vi "water_level_UI.vi"() -> ()   [LabVIEW 2020]
panel:
  out "Water level status":dbl(slide) scale=0.0..100.0
  in  "VISA resource name":refnum<visa-resource-name>
  in  "Table Control":string[][](table)
  out "Water level status":dbl(graph)
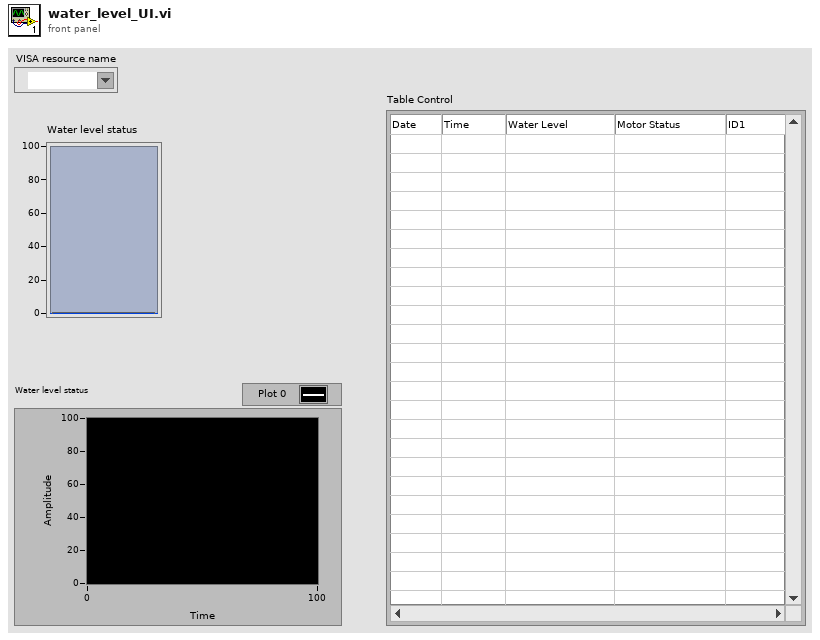
[diagram p1: front panel]
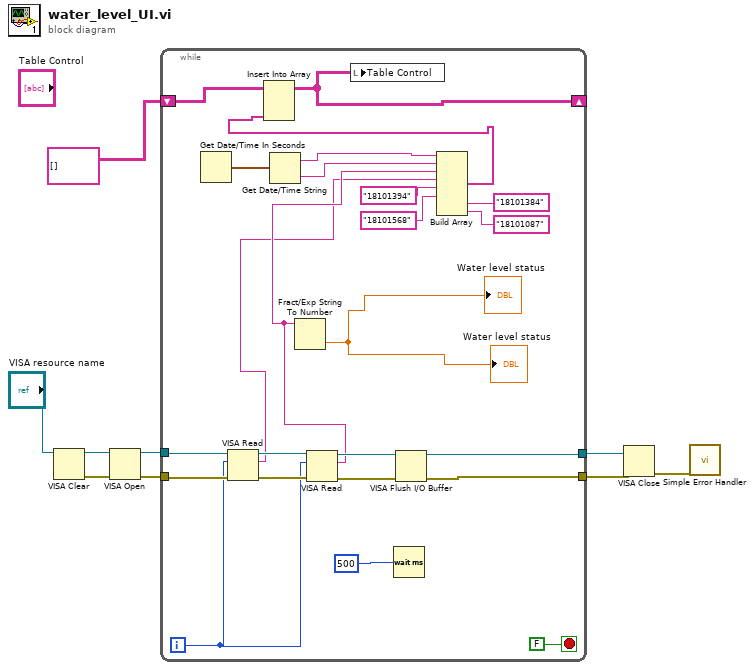
[diagram p0: block diagram]
diagram:
  n1 = VISA Clear(VISA resource name="VISA resource name") -> (VISA resource name out=w9:refnum<visa-resource-name>, error out=w8:errorcluster)  [unwired: 1 in]
  n2 = VISA Open(error in (no error)=w8, VISA resource name=w9) -> (VISA resource name=w7:refnum<visa-resource-name>, error out=w6:errorcluster)  [unwired: 3 in]
  n3 = while {
    tunnel: w7 -> [w33]
    tunnel: w6 -> [w32]
    tunnel: [w31] -> w5
    tunnel: [w30] -> w4
    shift-right: [w27] -> _
    shift-left: string[][] [] -> [w28]
    i -> [w12]
    stop <- FALSE stop-if-true
    n4 = Get Date/Time In Seconds() -> (seconds since 1Jan1904=w26:timestamp)
    n5 = VISA Read(VISA resource name=w33, byte count=w12, error in (no error)=w32) -> (VISA resource name out=w16:refnum<visa-resource-name>, read buffer=w10:string, error out=w15:errorcluster)  [unwired: 1 out]
    n6 = Get Date/Time String(seconds (now)=w26) -> (date string=w25:string, time string=w24:string)  [unwired: 2 in]
    n7 = VISA Read(VISA resource name=w16, byte count=w12, error in (no error)=w15) -> (VISA resource name out=w14:refnum<visa-resource-name>, read buffer=w11:string, error out=w13:errorcluster)  [unwired: 1 out]
    n8 = Fract/Exp String To Number(string=w11) -> (number=→"Water level status" →"Water level status":dbl)  [unwired: 3 in, 1 out]
    n9 = Wait (ms)(milliseconds to wait=u32 500) -> ()  [unwired: 1 out]
    n10 = VISA Flush I/O Buffer(VISA resource name=w14, error in (no error)=w13) -> (VISA resource name out=w31:refnum<visa-resource-name>, error out=w30:errorcluster)  [unwired: 1 in]
    n11 = Build Array(w25, w24, w11, w10, "18101394" ("element"), "18101568" ("element"), "18101384" ("element"), "18101087" ("element")) -> (w23:string[])
    n12 = Insert Into Array(array=w28, new element=w23) -> (w27:string[][])  [unwired: 2 in]
    n13 = local write "Table Control"(w27) -> ()
  }
  n14 = VISA Close(VISA resource name=w5, error in (no error)=w4) -> (error out=w3:errorcluster)
  n15 = call <vilib>:"Simple Error Handler.vi"("error in (no error)"=w3) -> ()  [unwired: 4 in, 5 out]
